vi "OP500Z8M_ReadFromPDU.vi"(8 "errin":errorcluster, 10 "SN":string, 11 "VISA ITECH Name ?":refnum<visa-resource-name>) -> (0 "errout":errorcluster, 2 "All Data":string[](array[string]), 3 "BMS OK ?":bool)   [LabVIEW 2020]
uses:
  <userlib>/PCAN Basic/Controls/BaudrateEenum.ctl
  <userlib>/PCAN Basic/Controls/Channel.ctl
  C:/Users/elhajj/OneDrive - FORSEE POWER/Bureau/Support banc de test/Ligne ZENPLUS/Code LabVIEW/CODE/02 SLIM ZEN WS 500/SubVi/FGV.ctl
  VG/VG_progressBar.vi
  <vilib>/Utility/file.llb/Write Delimited Spreadsheet (string).vi
  VG/VG_DCIRCurrent.vi
  VG/VG_DCIR+OUIouNON.vi
  <instrlib>/IT6000C/IT6000C.lvlib
  <userlib>/PCAN Basic/PCANBasic.lvlib
panel:
  out "Numeric":i32
  out "Stop":bool
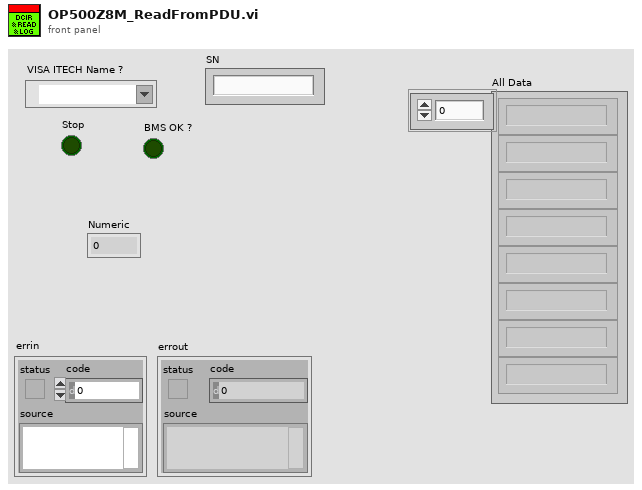
[diagram p1: front panel]
types:
  T1 = typedef "PCANBasic.lvlib/Channel.ctl" = enum16{"PCAN_NONEBUS", "not used1", "not used2", "not used3", "not used4", "not used5", "not used6", "not used7", "not used8", "not used9", "not used10", "not used11", "not used12", "not used13", "not used14", "not used15", "not used16", "not used17", "not used18", "not used19", "not used20", "not used21", "not used22", "not used23", "not used24", "not used25", "not used26", "not used27", "not used28", "not used29", "not used30", "not used31", "not used32", "PCAN_ISABUS1", "PCAN_ISABUS2", "PCAN_ISABUS3", "PCAN_ISABUS4", "PCAN_ISABUS5", "PCAN_ISABUS6", "PCAN_ISABUS7", "PCAN_ISABUS8", "not used41", "not used42", "not used43", "not used44", "not used45", "not used46", "not used47", "not used48", "PCAN_DNGBUS1", "not used50", "not used51", "not used52", "not used53", "not used54", "not used55", "not used56", "not used57", "not used58", "not used59", "not used60", "not used61", "not used62", "not used63", "not used64", "PCAN_PCIBUS1", "PCAN_PCIBUS2", "PCAN_PCIBUS3", "PCAN_PCIBUS4", "PCAN_PCIBUS5", "PCAN_PCIBUS6", "PCAN_PCIBUS7", "PCAN_PCIBUS8", "not used73", "not used74", "not used75", "not used76", "not used77", "not used78", "not used79", "not used80", "PCAN_USBBUS1", "PCAN_USBBUS2", "PCAN_USBBUS3", "PCAN_USBBUS4", "PCAN_USBBUS5", "PCAN_USBBUS6", "PCAN_USBBUS7", "PCAN_USBBUS8", "Not used89", "Not used90", "Not used91", "Not used92", "Not used93", "Not used94", "Not used95", "Not used96", "PCAN_PCCBUS1", "PCAN_PCCBUS2"}
  T2 = typedef "PCANBasic.lvlib/BaudrateEenum.ctl" = enum16{"CAN_Baud_1M", "CAN_Baud_800K", "CAN_BAUD_500K", "CAN_BAUD_250K", "CAN_BAUD_125K", "CAN_BAUD_100K", "CAN_BAUD_95K", "CAN_BAUD_83K", "CAN_BAUD_50K", "CAN_BAUD_47K", "CAN_BAUD_33K", "CAN_BAUD_20K", "CAN_BAUD_10K", "CAN_BAUD_5K", "User Baudrate"}
  T3 = typedef "FGV.ctl" = enum16{"GET", "SET", "RAZ"}
  T4 = typedef "PCANBasic.lvlib/CAN MSG Cluster.ctl" = cluster{"ID":u32, "MSG type":enum8{"STD", "RTR", "XTD", "XTD RTR", "STATUS"}, "LEN":i8, "DATA":u8[]}
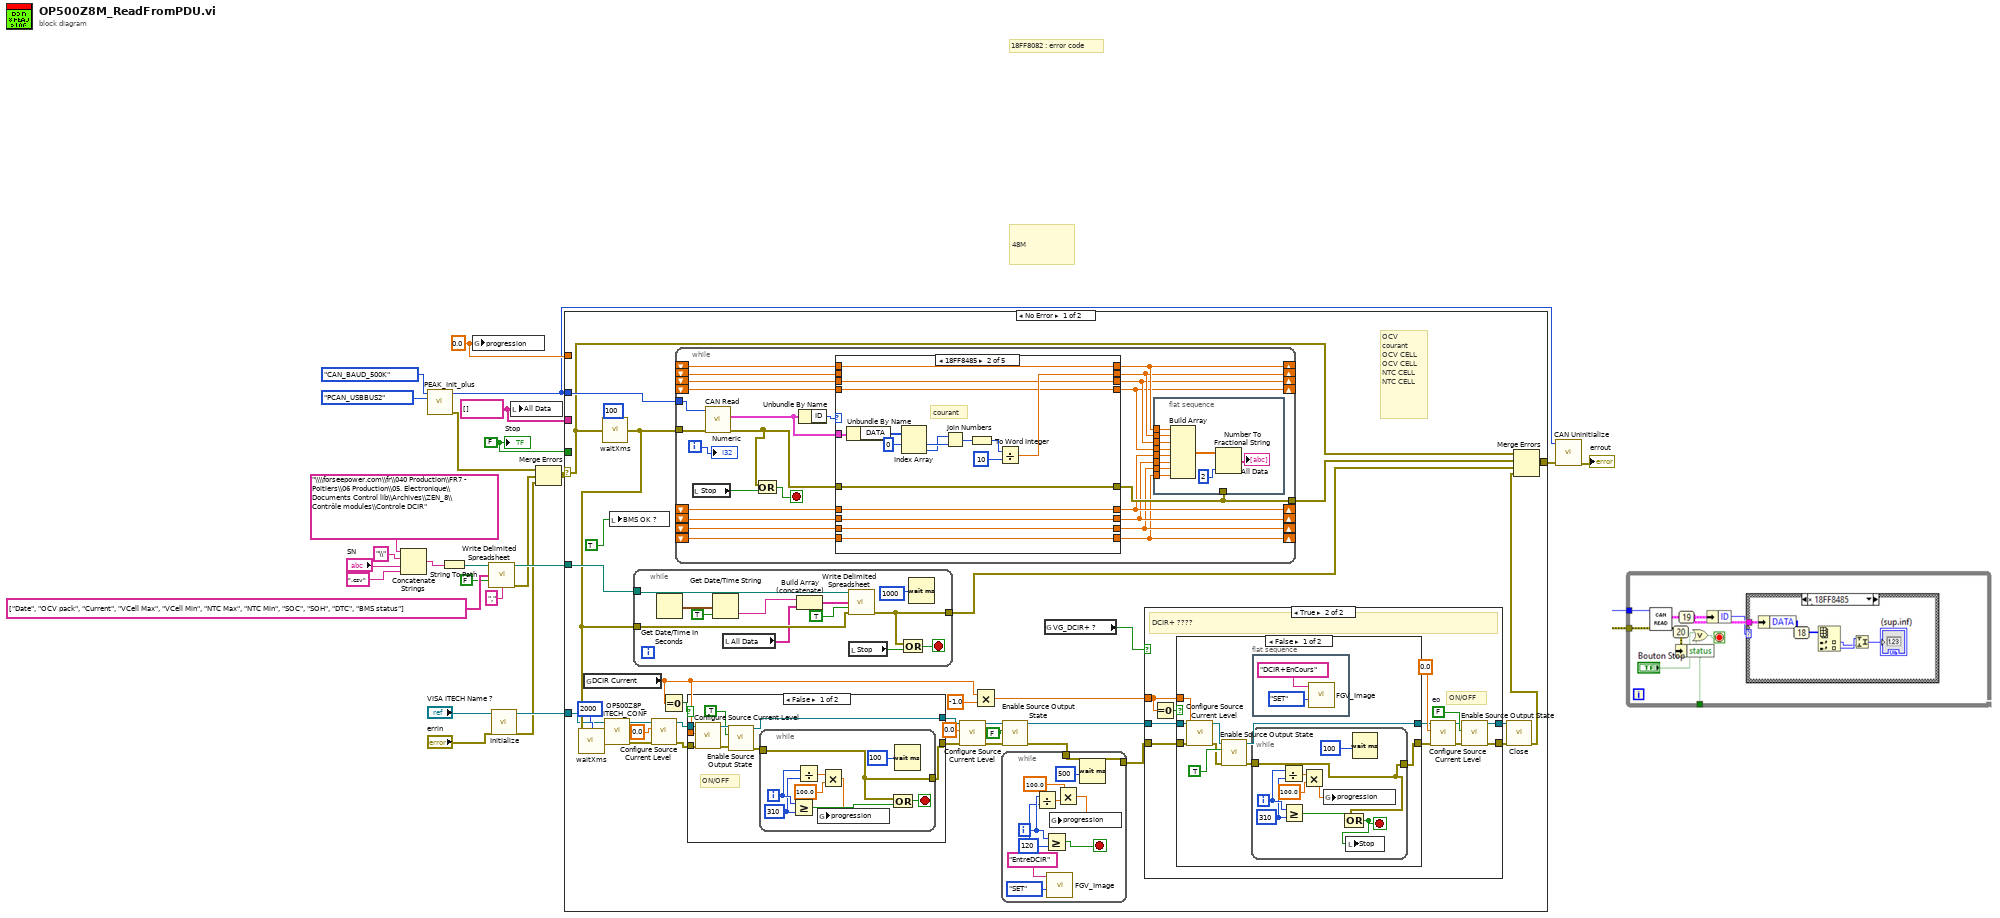
[diagram p0: block diagram]
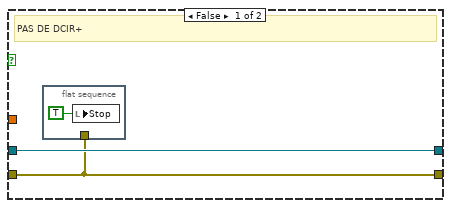
[diagram p3: hidden frame]
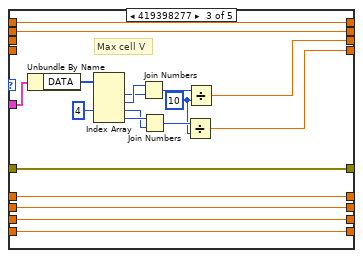
[diagram p6: hidden frame]
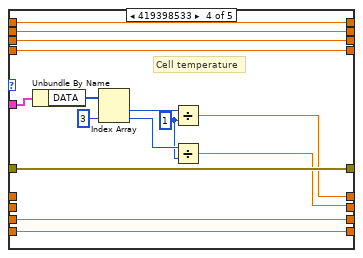
[diagram p7: hidden frame]
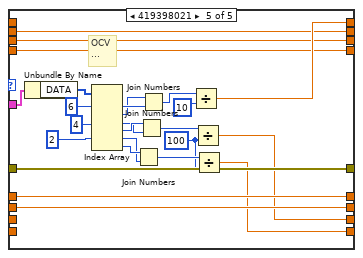
[diagram p8: hidden frame]
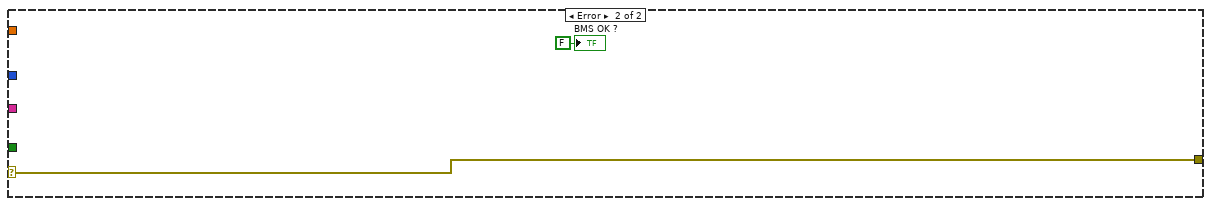
[diagram p9: hidden frame]
diagram:
  w8 = FALSE ("Stop")
  w19 = 0.0 ("progression")
  w20 = string[] []
  # "48M"
  # "18FF8082 : error code"
  n1 = Concatenate Strings("\\\\forseepower.com\\fr\\040 Production\\FR7 - Poitiers\\06 Production\\05. Electronique\\Documents Control lib\\Archives\\ZEN_8\\Contrôle modules\\Controle DCIR" ("chaîne"), "\\" ("chaîne"), "SN", ".csv" ("chaîne")) -> (w10:string)
  n2 = call <userlib>:"PEAK_Init_plus.vi"("Channel"=Channel."PCAN_USBBUS2", "BTR0BTR1"=BaudrateEenum."CAN_BAUD_500K") -> ("errout"=w1:errorcluster, "Channel out"=w2:T1)  [unwired: 8 in]
  n3 = String To Path(string=w10) -> (path=w11:path)
  n4 = global write "VG_progressBar.vi" "progression"(w19) -> ()
  n5 = call-poly <vilib>:"Write Delimited Spreadsheet.vi"("file path (dialog if empty)"=w11, "1D data"=string[] ["Date", "OCV pack", "Current", "VCell Max", "VCell Min", "NTC Max", "NTC Min", "SOC", "SOH", "DTC", "BMS status"], "append to file? (new file:F)"=FALSE, "delimiter (\\t)"="," ("delimiter (\\t)")) -> ("new file path (Not A Path if cancelled)"=w24:path, "error out"=w21:errorcluster)  [unwired: 10 in]
  n6 = call <instrlib>:"Initialize.vi"("error in (no error)"="errin", "VISA resource name"="VISA ITECH Name ?") -> ("error out"=w16:errorcluster, "VISA resource name out"=w17:refnum<visa-resource-name>)  [unwired: 8 in]
  n7 = local write "All Data"(w20) -> ()
  n8 = Merge Errors(w1, w21, w16) -> (w22:errorcluster)
  n9 = case shown="No Error" w22 {
    selector: w22 -> [w50 w261]
    tunnel: [w59 w261] -> w6
    tunnel: w24 -> [w53 _]
    tunnel: w20 -> [_ _]
    tunnel: w19 -> [_ _]
    tunnel: w17 -> [w36 _]
    tunnel: w8 -> [_ _]
    tunnel: w2 -> [w51 _]
    frame No Error {
      # "OCV\ncourant\nOCV CELL\nOCV CELL\nNTC CELL\nNTC CELL"
      n10 = global read "VG_DCIRCurrent.vi" "DCIR Current"() -> (w32:dbl)
      n11 = call <userlib>:"waitXms.vi"("attente (ms)"=u32 100, "errin"=w50) -> ("errout"=w43:errorcluster)  [unwired: 13 in]
      n12 = call <userlib>:"waitXms.vi"("attente (ms)"=u32 2000, "errin"=w43) -> ("errout"=w38:errorcluster)  [unwired: 13 in]
      n13 = call "OP500Z8P_ITECH_CONF.vi"("ErrIN"=w38, "VISAin"=w36) -> ("ErrOUT"=w37:errorcluster, "VisaOUT"=w35:refnum<visa-resource-name>)  [unwired: 8 in]
      n14 = local write "BMS OK ?"(TRUE ("BMS OK ?")) -> ()
      n15 = while {
        tunnel: w53 -> [w254]
        tunnel: w43 -> [w253]
        tunnel: [w248] -> w45
        stop <- w250 stop-if-true
        n16 = Get Date/Time In Seconds() -> (seconds since 1Jan1904=w258:timestamp)
        n17 = Get Date/Time String(seconds (now)=w258, want seconds? (F)=TRUE ("secondes ? (F)")) -> (time string=w252:string)  [unwired: 1 in, 1 out]
        n18 = local read "All Data"() -> (w251:string[])
        n19 = Build Array (concatenate)(w252, w251) -> (w256:string[])
        n20 = call-poly <vilib>:"Write Delimited Spreadsheet.vi"("file path (dialog if empty)"=w254, "1D data"=w256, "append to file? (new file:F)"=TRUE, "error in (no error)"=w253) -> ("error out"=w248:errorcluster)  [unwired: 10 in, 1 out]
        n21 = local read "Stop"() -> (w249:bool)
        n22 = Compound Arithmetic op=OR ("Opérateur arithmétique")(w248, w249) -> (w250:bool)
        n23 = Wait (ms)(milliseconds to wait=u32 1000 ("attente (ms)")) -> ()  [unwired: 1 out]
      }
      n24 = call <instrlib>:"Configure Source Current Level.vi"("error in (no error)"=w37, "Value(0)"=0.0, "VISA resource name"=w35) -> ("error out"=w33:errorcluster, "VISA resource name out"=w34:refnum<visa-resource-name>)  [unwired: 7 in]
      n25 = Equal To 0?(x=w32) -> (x = 0?=w31:bool)
      n26 = while {
        tunnel: w43 -> [w151]
        tunnel: [w148] -> w52
        tunnel: w51 -> [w145]
        shift-right: [w141] -> _
        shift-left: _ -> [w142]
        shift-right: [w139] -> _
        shift-left: _ -> [w140]
        shift-right: [w138] -> _
        shift-left: _ -> [w136]
        shift-right: [w137] -> _
        shift-left: _ -> [w135]
        shift-right: [w132] -> _
        shift-left: _ -> [w134]
        shift-right: [w131] -> _
        shift-left: _ -> [w133]
        shift-right: [w130] -> _
        shift-left: _ -> [w129]
        shift-right: [w127] -> _
        shift-left: _ -> [w128]
        i -> [w144]
        stop <- w146 stop-if-true
        n27 = local read "Stop"() -> (w143:bool)
        n28 = call <userlib>:"CAN Read.vi"("error in (no error)"=w151, "Channel"=w145) -> ("error out"=w147:errorcluster, "CAN_Message out"=w149:T4)  [unwired: 5 in, 3 out]
        n29 = Compound Arithmetic op=OR ("Opérateur arithmétique")(w147, w143) -> (w146:bool)
        n30 = Unbundle By Name(w149) -> ("ID"=w150:u32)
        n31 = case shown="18FF8485" w150 {
          tunnel: w149 -> [_ w186 w204 w219 w246]
          tunnel: w147 -> [w170 w187 w206 w222 w247]
          tunnel: [w170 w187 w206 w222 w247] -> w148
          tunnel: [w171 w188 w207 w221 w239] -> w141
          tunnel: w142 -> [w171 w188 w207 w221 _]
          tunnel: [w169 w178 w203 w218 w238] -> w139
          tunnel: w140 -> [w169 _ w203 w218 w238]
          tunnel: [w168 w177 w199 w217 w237] -> w138
          tunnel: [w167 w176 w193 w216 w236] -> w137
          tunnel: w136 -> [w168 w177 _ w217 w237]
          tunnel: w135 -> [w167 w176 _ w216 w236]
          tunnel: [w166 w175 w192 w214 w235] -> w132
          tunnel: [w165 w174 w191 w210 w234] -> w131
          tunnel: w134 -> [w166 w175 w192 _ w235]
          tunnel: w133 -> [w165 w174 w191 _ w234]
          tunnel: [w164 w173 w190 w209 w229] -> w130
          tunnel: [w163 w172 w189 w208 w223] -> w127
          tunnel: w129 -> [w164 w173 w190 w209 _]
          tunnel: w128 -> [w163 w172 w189 w208 _]
          frame 0, Default {
          }
          frame 419398789 {
            # "courant"
            n32 = Unbundle By Name(w186) -> ("DATA"=w185:u8[])
            n33 = Index Array(array=w185, index #1=0 ("index")) -> (element #1=w183:u8, element #2=w182:u8)  [unwired: 1 in]
            n34 = Join Numbers(hi=w182, lo=w183) -> ((hi.lo)=w181:u16)
            n35 = To Word Integer(number=w181) -> (16bit integer=w180:i16)
            n36 = Divide(x=w180, y=i16 10) -> (x/y=w178:dbl)
          }
          frame 419398277 {
            w194 = u16 10 ("y")
            # "Max cell V"
            n37 = Unbundle By Name(w204) -> ("DATA"=w205:u8[])
            n38 = Index Array(array=w205, index #3=4 ("index")) -> (element #1=w201:u8, element #2=w202:u8, element #3=w196:u8, element #4=w197:u8)  [unwired: 3 in]
            n39 = Join Numbers(hi=w202, lo=w201) -> ((hi.lo)=w200:u16)
            n40 = Join Numbers(hi=w197, lo=w196) -> ((hi.lo)=w195:u16)
            n41 = Divide(x=w195, y=w194) -> (x/y=w193:dbl)
            n42 = Divide(x=w200, y=w194) -> (x/y=w199:dbl)
          }
          frame 419398533 {
            w211 = u8 1 ("y")
            # "Cell temperature"
            n43 = Unbundle By Name(w219) -> ("DATA"=w220:u8[])
            n44 = Index Array(array=w220, index #2=3 ("index")) -> (element #1=w215:u8, element #2=w212:u8)  [unwired: 1 in]
            n45 = Divide(x=w215, y=w211) -> (x/y=w214:dbl)
            n46 = Divide(x=w212, y=w211) -> (x/y=w210:dbl)
          }
          frame 419398021 {
            w224 = u16 100 ("y")
            # "OCV\n..."
            n47 = Unbundle By Name(w246) -> ("DATA"=w245:u8[])
            n48 = Index Array(array=w245, index #1=6 ("index"), index #3=4 ("index"), index #5=2 ("index")) -> (element #1=w243:u8, element #2=w242:u8, element #3=w231:u8, element #4=w232:u8, element #5=w227:u8, element #6=w228:u8)  [unwired: 3 in]
            n49 = Join Numbers(hi=w228, lo=w227) -> ((hi.lo)=w225:u16)
            n50 = Join Numbers(hi=w232, lo=w231) -> ((hi.lo)=w230:u16)
            n51 = Join Numbers(hi=w242, lo=w243) -> ((hi.lo)=w241:u16)
            n52 = Divide(x=w241, y=u16 10) -> (x/y=w239:dbl)
            n53 = Divide(x=w230, y=w224) -> (x/y=w229:dbl)
            n54 = Divide(x=w225, y=w224) -> (x/y=w223:dbl)
          }
        }
        n55 = flat-sequence {
          tunnel: w148 -> [_]
          tunnel: w141 -> [w159]
          tunnel: w139 -> [w158]
          tunnel: w138 -> [w157]
          tunnel: w137 -> [w156]
          tunnel: w132 -> [w155]
          tunnel: w131 -> [w154]
          tunnel: w130 -> [w153]
          tunnel: w127 -> [w152]
          frame #0 {
            n56 = Build Array(w159, w158, w157, w156, w155, w154, w153, w152) -> (w162:dbl[])
            n57 = Number To Fractional String(number=w162, precision (6)=i16 2 ("précision (6)")) -> (F-format string=→"All Data":string[])  [unwired: 2 in]
          }
        }
        "Numeric" <- w144
      }
      n58 = case shown="False" w31 {
        tunnel: w34 -> [w74 w89]
        tunnel: w33 -> [w73 w88]
        tunnel: w32 -> [w72 _]
        tunnel: [w71 w89] -> w30
        tunnel: [w70 w88] -> w29
        frame False {
          # "ON/OFF"
          n59 = call <instrlib>:"Configure Source Current Level.vi"("error in (no error)"=w73, "Value(0)"=w72, "VISA resource name"=w74) -> ("error out"=w78:errorcluster, "VISA resource name out"=w77:refnum<visa-resource-name>)  [unwired: 7 in]
          n60 = call <instrlib>:"Enable Source Output State.vi"("error in (no error)"=w78, "Enable(True)"=TRUE, "VISA resource name"=w77) -> ("error out"=w75:errorcluster, "VISA resource name out"=w71:refnum<visa-resource-name>)  [unwired: 7 in]
          n61 = while {
            tunnel: w75 -> [w79]
            tunnel: [w79] -> w70
            i -> [w85]
            stop <- w80 stop-if-true
            w84 = 310 ("y")
            n62 = Greater Or Equal?(x=w85, y=w84) -> (x >= y?=w86:bool)
            n63 = Divide(x=w85, y=w84) -> (x/y=w83:dbl)
            n64 = Multiply(x=w83, y=100.0) -> (x*y=w81:dbl)
            n65 = global write "VG_progressBar.vi" "progression"(w81) -> ()
            n66 = Compound Arithmetic op=OR ("Opérateur arithmétique")(w79, w86) -> (w80:bool)
            n67 = Wait (ms)(milliseconds to wait=u32 100 ("attente (ms)")) -> ()  [unwired: 1 out]
          }
        }
        frame True {
        }
      }
      n68 = call <instrlib>:"Configure Source Current Level.vi"("error in (no error)"=w29, "Value(0)"=0.0, "VISA resource name"=w30) -> ("error out"=w41:errorcluster, "VISA resource name out"=w40:refnum<visa-resource-name>)  [unwired: 7 in]
      n69 = Multiply(x=w32, y=-1.0) -> (x*y=w47:dbl)
      n70 = call <instrlib>:"Enable Source Output State.vi"("error in (no error)"=w41, "Enable(True)"=FALSE, "VISA resource name"=w40) -> ("error out"=w27:errorcluster, "VISA resource name out"=w39:refnum<visa-resource-name>)  [unwired: 7 in]
      n71 = while {
        tunnel: w27 -> [w60]
        tunnel: [w60] -> w26
        i -> [w67]
        stop <- w68 stop-if-true
        w66 = 120 ("y")
        n72 = Divide(x=w67, y=w66) -> (x/y=w65:dbl)
        n73 = Greater Or Equal?(x=w67, y=w66) -> (x >= y?=w68:bool)
        n74 = call "FGV_Image.vi"("Énum"=FGV."SET", "IN"="EntreDCIR") -> ()  [unwired: 9 in, 1 out]
        n75 = Multiply(x=100.0, y=w65) -> (x*y=w63:dbl)
        n76 = global write "VG_progressBar.vi" "progression"(w63) -> ()
        n77 = Wait (ms)(milliseconds to wait=u32 500 ("attente (ms)")) -> ()  [unwired: 1 out]
      }
      n78 = global read "VG_DCIR+OUIouNON.vi" "VG_DCIR+ ?"() -> (w28:bool)
      n79 = case shown="True" w28 {
        tunnel: [w90 w100] -> w57
        tunnel: [w91 w99] -> w56
        tunnel: w47 -> [_ w95]
        tunnel: w26 -> [w90 w93]
        tunnel: w39 -> [w91 w97]
        frame False {
          # "PAS DE DCIR+"
          n80 = flat-sequence {
            tunnel: w90 -> [_]
            frame #0 {
              n81 = local write "Stop"(TRUE ("Stop")) -> ()
            }
          }
        }
        frame True {
          w104 = FALSE  # eo
          # "ON/OFF"
          # "DCIR+ ????"
          n82 = Equal To 0?(x=w95) -> (x = 0?=w94:bool)
          n83 = case shown="False" w94 {
            tunnel: [w105 w126] -> w98
            tunnel: w95 -> [w111 _]
            tunnel: w97 -> [w112 w126]
            tunnel: [w109 w125] -> w96
            tunnel: w93 -> [w113 w125]
            frame False {
              n84 = call <instrlib>:"Configure Source Current Level.vi"("error in (no error)"=w113, "Value(0)"=w111, "VISA resource name"=w112) -> ("error out"=w108:errorcluster, "VISA resource name out"=w106:refnum<visa-resource-name>)  [unwired: 7 in]
              n85 = call <instrlib>:"Enable Source Output State.vi"("error in (no error)"=w108, "Enable(True)"=TRUE, "VISA resource name"=w106) -> ("error out"=w107:errorcluster, "VISA resource name out"=w105:refnum<visa-resource-name>)  [unwired: 7 in]
              n86 = while {
                tunnel: w107 -> [w116]
                tunnel: [w116] -> w109
                i -> [w120]
                stop <- w117 stop-if-true
                w119 = u32 310 ("attente (ms)")
                n87 = Divide(x=w120, y=w119) -> (x/y=w122:dbl)
                n88 = Greater Or Equal?(x=w120, y=w119) -> (x >= y?=w123:bool)
                n89 = Multiply(x=w122, y=100.0) -> (x*y=w118:dbl)
                n90 = global write "VG_progressBar.vi" "progression"(w118) -> ()
                n91 = Compound Arithmetic op=OR ("Opérateur arithmétique")(w116, w123) -> (w117:bool)
                n92 = local write "Stop"(w117) -> ()
                n93 = Wait (ms)(milliseconds to wait=u32 100 ("attente (ms)")) -> ()  [unwired: 1 out]
              }
              n94 = flat-sequence {
                frame #0 {
                  n95 = call "FGV_Image.vi"("Énum"=FGV."SET", "IN"="DCIR+EnCours") -> ()  [unwired: 9 in, 1 out]
                }
              }
            }
            frame True {
            }
          }
          n96 = call <instrlib>:"Configure Source Current Level.vi"("error in (no error)"=w96, "Value(0)"=0.0, "VISA resource name"=w98) -> ("error out"=w103:errorcluster, "VISA resource name out"=w102:refnum<visa-resource-name>)  [unwired: 7 in]
          n97 = call <instrlib>:"Enable Source Output State.vi"("error in (no error)"=w103, "Enable(True)"=w104, "VISA resource name"=w102) -> ("error out"=w100:errorcluster, "VISA resource name out"=w99:refnum<visa-resource-name>)  [unwired: 7 in]
        }
      }
      n98 = call <instrlib>:"Close.vi"("error in (no error)"=w57, "VISA resource name"=w56) -> ("error out"=w55:errorcluster)  [unwired: 9 in]
      n99 = Merge Errors(w50, w52, w45, w55) -> (w59:errorcluster)
    }
    frame Error {
      "BMS OK ?" <- FALSE ("BMS OK ?")
    }
  }
  n100 = call <userlib>:"CAN Uninitialize.vi"("error in (no error)"=w6, "Channel"=w2) -> ("error out"=→"errout":errorcluster)  [unwired: 7 in, 2 out]
  "Stop" <- w8
